vi "InstanceDestroy.vi"(8 "error in (no error)":errorcluster, 11 "Singleton.lvclass In":refnum<class "Singleton.lvclass">) -> (0 "error out":errorcluster, 3 "Singleton.lvclass Out":refnum<class "Singleton.lvclass">)   [LabVIEW 2013, in "Singleton.lvclass"]
uses:
  Singleton.lvclass
panel:
  # "SingletonInstance\nDestroy"
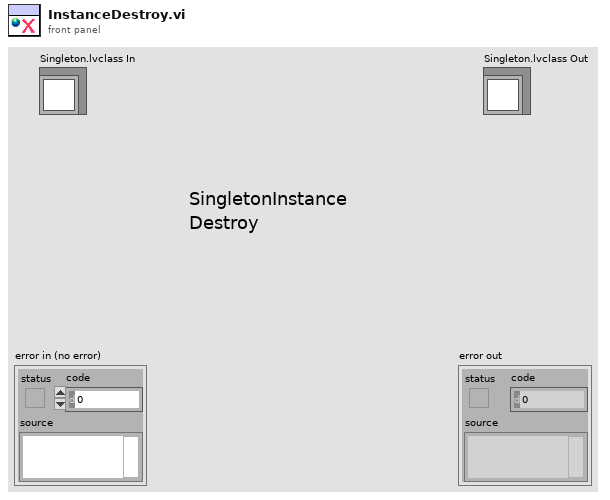
[diagram p1: front panel]
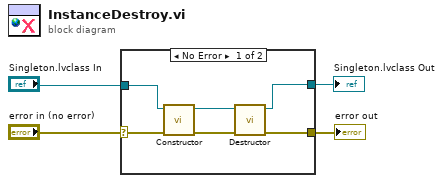
[diagram p0: block diagram]
diagram:
  n1 = case shown="No Error" "error in (no error)" {
    selector: "error in (no error)" -> [w8 w12]
    tunnel: [w7 w12] -> w3
    tunnel: "Singleton.lvclass In" -> [w6 w11]
    tunnel: [w5 w11] -> w1
    frame No Error {
      n2 = call "Constructor.vi"("error in (no error)"=w8, "Singleton.lvclass In"=w6) -> ("error out"=w9:errorcluster, "SingletonDVR Out"=w10:refnum<data-value>)  [unwired: 8 in]
      n3 = call "Destructor.vi"("error in (no error)"=w9, "SingletonDVR In"=w10) -> ("error out"=w7:errorcluster, "Singleton.lvclass Out"=w5:refnum<class "Singleton.lvclass">)  [unwired: 8 in]
    }
    frame Error {
    }
  }
  "error out" <- w3
  "Singleton.lvclass Out" <- w1
